vi "motor_block2.vi"(8 "error in":errorcluster, 10 "unit ID":u8, 11 "Modbus master in":refnum<class "Modbus Master.lvclass">) -> (0 "error out":errorcluster, 3 "Modbus master out":refnum<class "Modbus Master.lvclass">)   [LabVIEW 2020]
uses:
  <vilib>/NI/Modbus Library/API/Master/Modbus Master.lvclass
  C:/Program Files/National Instruments/LabVIEW 2020/vi.lib/NI/Modbus Library/API/Modbus API.lvclass
  <vilib>/NI/Modbus Library/API/Modbus API.lvclass/Modbus API.ctl
  <vilib>/NI/Modbus Library/Transmission Data Unit/Transmission Data Unit.lvclass/Transmission Data Unit.ctl
  <vilib>/NI/Modbus Library/Transmission Data Unit/Write Unit ID.vi
  <vilib>/NI/Modbus Library/API/Read Transmission Data Unit.vi
  <vilib>/NI/Modbus Library/API/Write Transmission Data Unit.vi
  status/emergency stop.vi
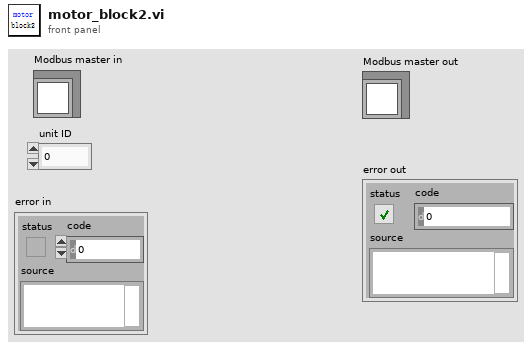
[diagram p1: front panel]
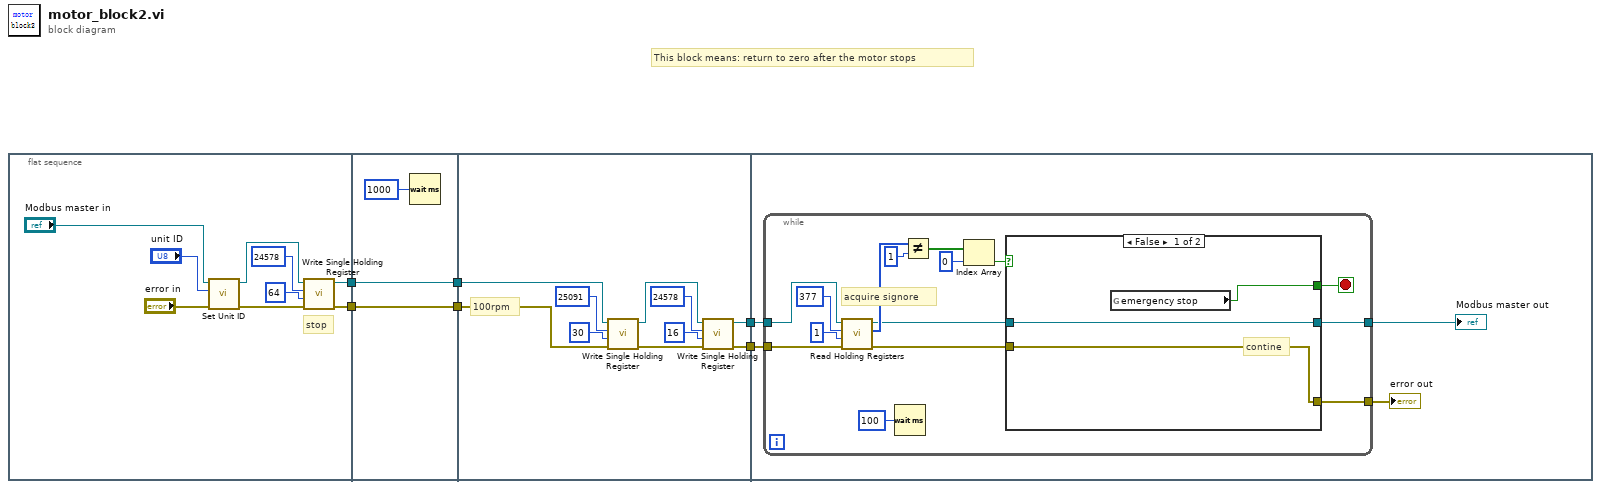
[diagram p0: block diagram]
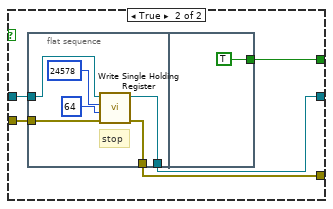
[diagram p2: hidden frame]
diagram:
  # "This block means: return to zero after the motor stops"
  n1 = flat-sequence {
    tunnel: [w10] -> w1
    tunnel: [w9] -> w2
    tunnel: w2 -> [w18]
    tunnel: [w18] -> w6
    tunnel: w1 -> [w17]
    tunnel: [w17] -> w5
    tunnel: w6 -> [w22]
    tunnel: w5 -> [w21]
    tunnel: [w20] -> w4
    tunnel: [w19] -> w3
    tunnel: w4 -> [w32]
    tunnel: w3 -> [w31]
    frame #0 {
      # "stop"
      n2 = call <vilib>:"Set Unit ID.vi"("error in"="error in", "unit ID"="unit ID", "Modbus master in"="Modbus master in") -> ("error out"=w7:errorcluster, "Modbus master out"=w8:refnum<class "Modbus Master.lvclass">)  [unwired: 7 in]
      n3 = call-dynamic "Write Single Holding Register.vi"("error in"=w7, "register to write"=u16 64 ("address"), "address"=u16 24578, "Modbus master in"=w8) -> ("error out"=w10:errorcluster, "Modbus master out"=w9:refnum<class "Modbus Master.lvclass">)  [unwired: 6 in]
    }
    frame #1 {
      n4 = Wait (ms)(milliseconds to wait=u32 1000) -> ()  [unwired: 1 out]
    }
    frame #2 {
      # "100rpm"
      n5 = call-dynamic "Write Single Holding Register.vi"("error in"=w21, "register to write"=u16 30 ("address"), "address"=u16 25091, "Modbus master in"=w22) -> ("error out"=w23:errorcluster, "Modbus master out"=w24:refnum<class "Modbus Master.lvclass">)  [unwired: 6 in]
      n6 = call-dynamic "Write Single Holding Register.vi"("error in"=w23, "register to write"=u16 16 ("address"), "address"=u16 24578, "Modbus master in"=w24) -> ("error out"=w19:errorcluster, "Modbus master out"=w20:refnum<class "Modbus Master.lvclass">)  [unwired: 6 in]
    }
    frame #3 {
      n7 = while {
        tunnel: [w38] -> w30
        tunnel: [w37] -> w29
        tunnel: w32 -> [w36]
        tunnel: w31 -> [w35]
        stop <- w39 stop-if-true
        # "acquire signore"
        n8 = call-dynamic "Read Holding Registers.vi"("error in"=w35, "number of inputs"=u16 1 ("address"), "starting address"=u16 377 ("address"), "Modbus master in"=w36) -> ("error out"=w40:errorcluster, "register values"=w46:u16[], "Modbus master out"=w41:refnum<class "Modbus Master.lvclass">)  [unwired: 5 in]
        n9 = Wait (ms)(milliseconds to wait=u32 100) -> ()  [unwired: 1 out]
        n10 = Not Equal?(x=w46, y=u16 1 ("number of inputs")) -> (x != y?=w44:bool[])
        n11 = Index Array(array=w44, index=0) -> (element=w42:bool)
        n12 = case shown="False" w42 {
          tunnel: w41 -> [w50 w55]
          tunnel: w40 -> [w49 w54]
          tunnel: [w48 w53] -> w39
          tunnel: [w50 w52] -> w38
          tunnel: [w49 w51] -> w37
          frame False {
            # "contine"
            n13 = global read "emergency stop.vi" "emergency stop"() -> (w48:bool)
          }
          frame True {
            n14 = flat-sequence {
              tunnel: w55 -> [w59]
              tunnel: w54 -> [w58]
              tunnel: [w57] -> w52
              tunnel: [w56] -> w51
              tunnel: [TRUE] -> w53
              frame #0 {
                # "stop"
                n15 = call-dynamic "Write Single Holding Register.vi"("error in"=w58, "register to write"=u16 64 ("address"), "address"=u16 24578, "Modbus master in"=w59) -> ("error out"=w56:errorcluster, "Modbus master out"=w57:refnum<class "Modbus Master.lvclass">)  [unwired: 6 in]
              }
              frame #1 {
              }
            }
          }
        }
      }
      "Modbus master out" <- w30
      "error out" <- w29
    }
  }
